vi "外观 1.vi"(0 "Data In":T6=enum."氨氮" caption="数据输入", 2 "Display State In":T3={"模块启用"={"环境动力"=FALSE, "氨氮"=FALSE, "总磷"=FALSE, "总氮"=FALSE, "高锰酸盐指数"=FALSE, "化学需氧量"=FALSE, "多参数"=FALSE, "加标回收"=FALSE, "GPS"=FALSE}, "模块名称"={"环境动力"="环境动力", "氨氮"="氨氮", "总磷"="总磷", "总氮"="总氮", "高锰酸盐指数"="高锰酸盐指数", "化学需氧量"="化学需氧量", "多参数"="多参数", "加标回收"="加标回收", "GPS"="GPS"}} caption="显示状态输入", 3 "Container State":T5 caption="容器状态") -> (6 "Data Out":T6=enum."氨氮" caption="数据输出", 7 "Display State Out":T3={"模块启用"={"环境动力"=FALSE, "氨氮"=FALSE, "总磷"=FALSE, "总氮"=FALSE, "高锰酸盐指数"=FALSE, "化学需氧量"=FALSE, "多参数"=FALSE, "加标回收"=FALSE, "GPS"=FALSE}, "模块名称"={"环境动力"="环境动力", "氨氮"="氨氮", "总磷"="总磷", "总氮"="总氮", "高锰酸盐指数"="高锰酸盐指数", "化学需氧量"="化学需氧量", "多参数"="多参数", "加标回收"="加标回收", "GPS"="GPS"}} caption="显示状态输出", 8 "Action":T2 caption="动作")   [LabVIEW 2016, in "运维调试菜单.xctl"]
uses:
  <vilib>/_xctls/Container State.ctl
  <vilib>/_xctls/Action.ctl
  <vilib>/Utility/miscctls.llb/LVPointTypeDef.ctl
  <vilib>/_xctls/XControlSupport.lvlib
panel:
  in  "单选按钮":T1
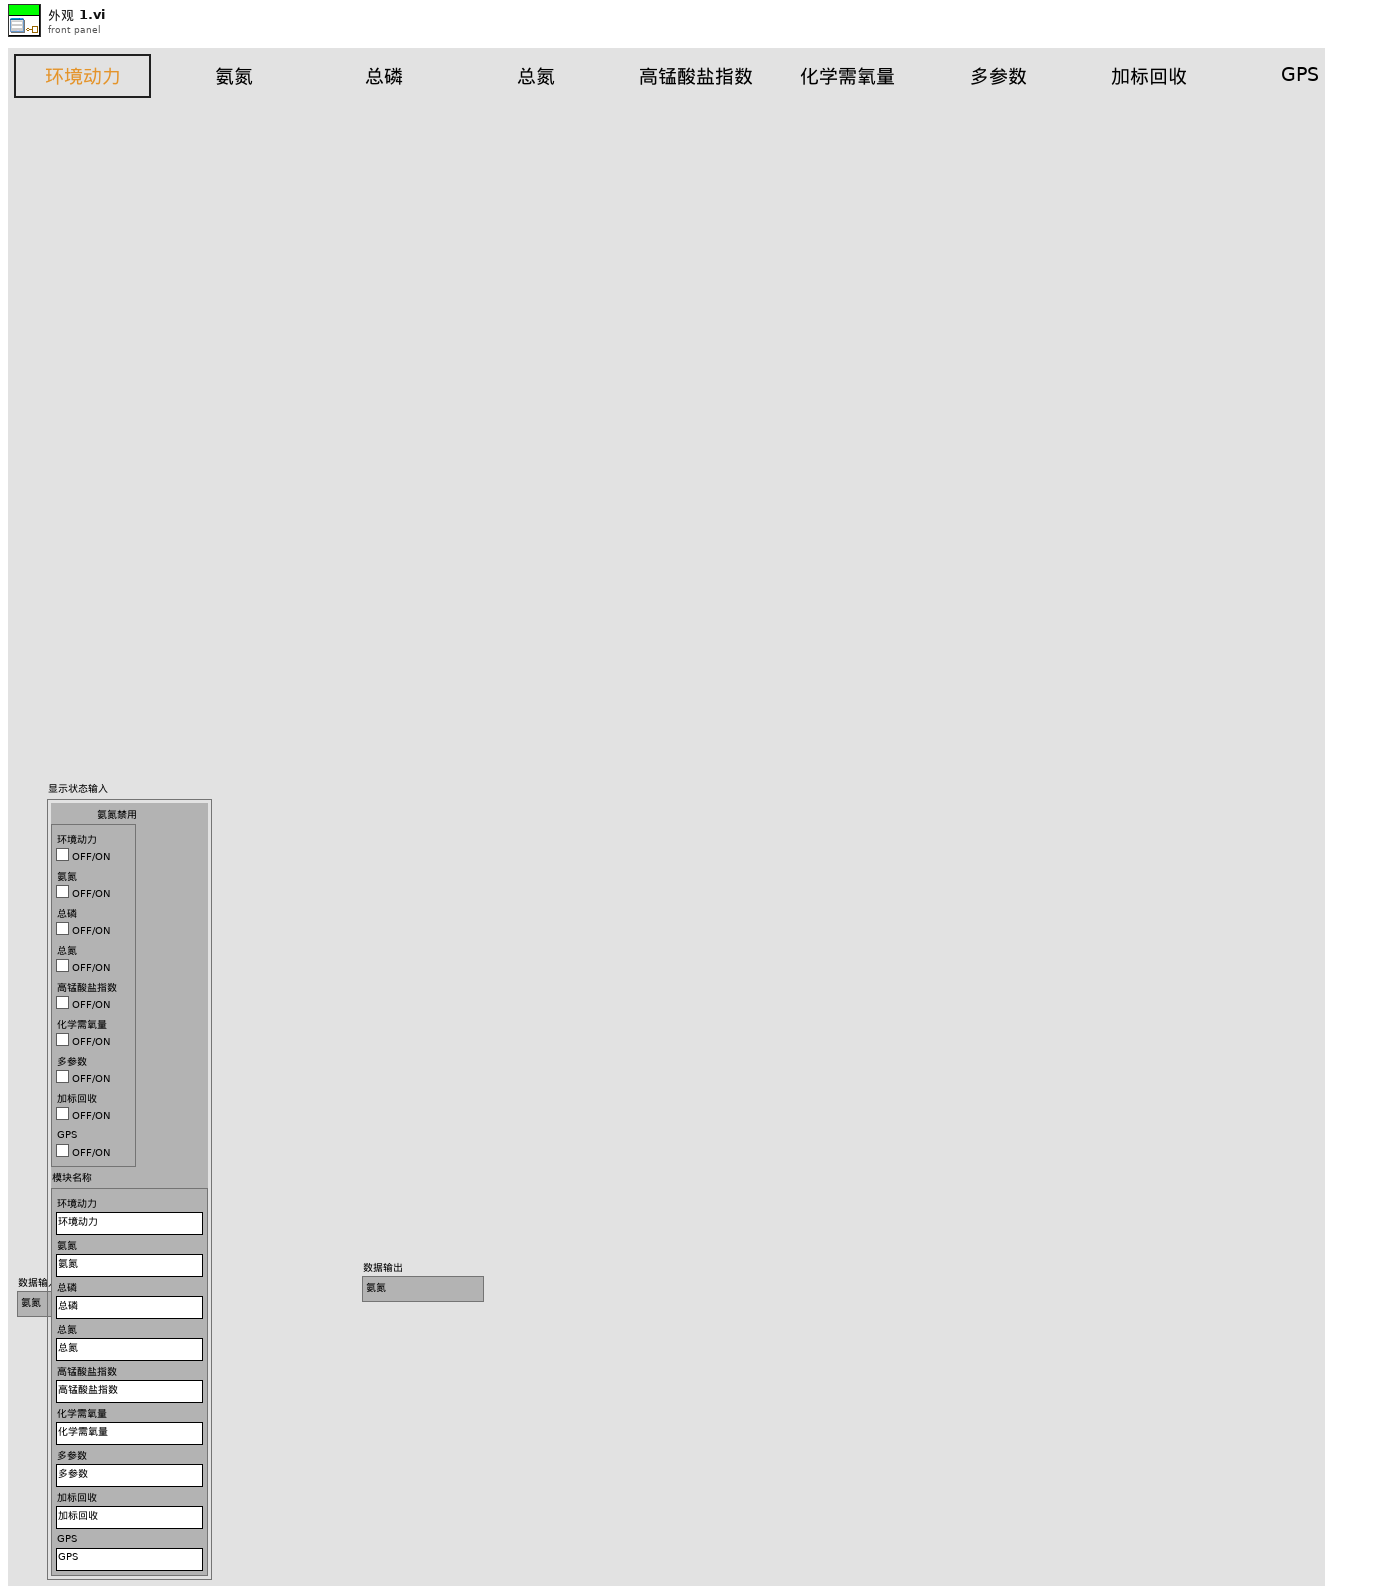
[diagram p1: front panel]
types:
  T1 = typedef "运维调试菜单.xctl/控件外观.ctl" = enum32{"环境动力", "氨氮", "总磷", "总氮", "高锰酸盐指数", "化学需氧量", "多参数", "加标回收", "GPS"}
  T2 = typedef "XControlSupport.lvlib/Action.ctl" = cluster{"Data Changed?":bool, "State Changed?":bool, "Action Name":string}
  T3 = typedef "运维调试菜单.xctl/状态 1.ctl" = cluster{"模块启用":T4, "模块名称":cluster{"环境动力":string, "氨氮":string, "总磷":string, "总氮":string, "高锰酸盐指数":string, "化学需氧量":string, "多参数":string, "加标回收":string, "GPS":string}}
  T4 = typedef "运维调试菜单.xctl/模块启用.ctl" = cluster{"环境动力":bool, "氨氮":bool, "总磷":bool, "总氮":bool, "高锰酸盐指数":bool, "化学需氧量":bool, "多参数":bool, "加标回收":bool, "GPS":bool}
  T5 = typedef "XControlSupport.lvlib/Container State.ctl" = cluster{"Indicator?":bool, "Run Mode?":bool, " Refnum":refnum<vi>}
  T6 = typedef "运维调试菜单.xctl/数据 1.ctl" = enum16{"环境动力", "氨氮", "总磷", "总氮", "高锰酸盐指数", "化学需氧量", "多参数", "加标回收", "GPS"}
  T7 = typedef "LVPointTypeDef.ctl" = cluster{"Horizontal":i16, "Vertical":i16}
  T8 = cluster{"环境动力":string, "氨氮":string, "总磷":string, "总氮":string, "高锰酸盐指数":string, "化学需氧量":string, "多参数":string, "加标回收":string, "GPS":string}
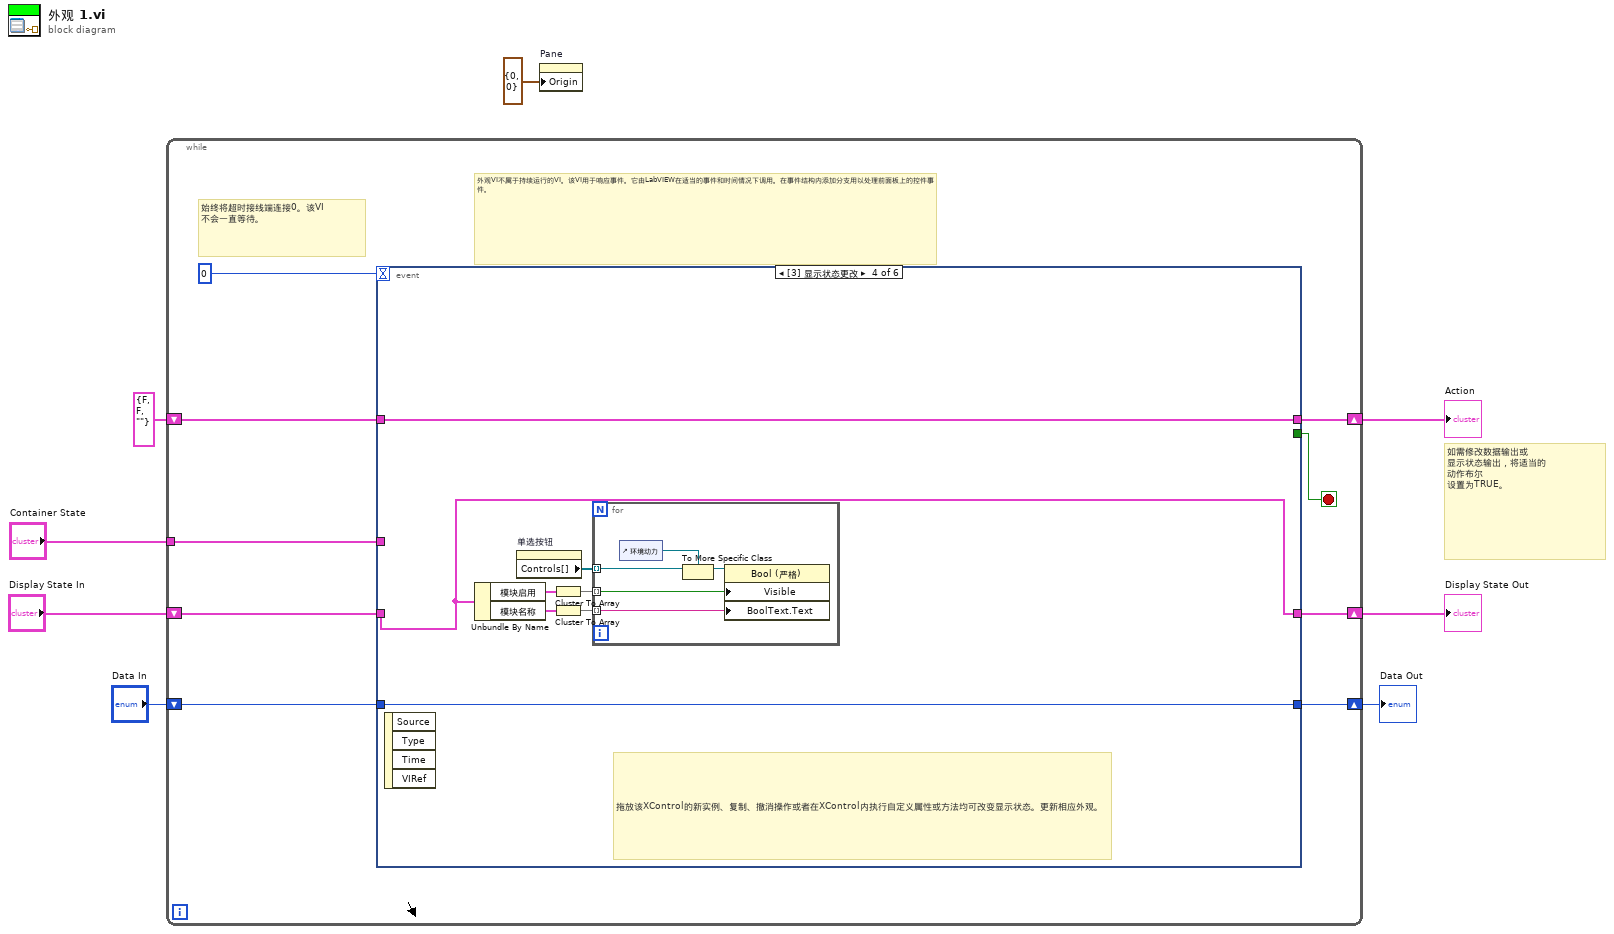
[diagram p0: block diagram]
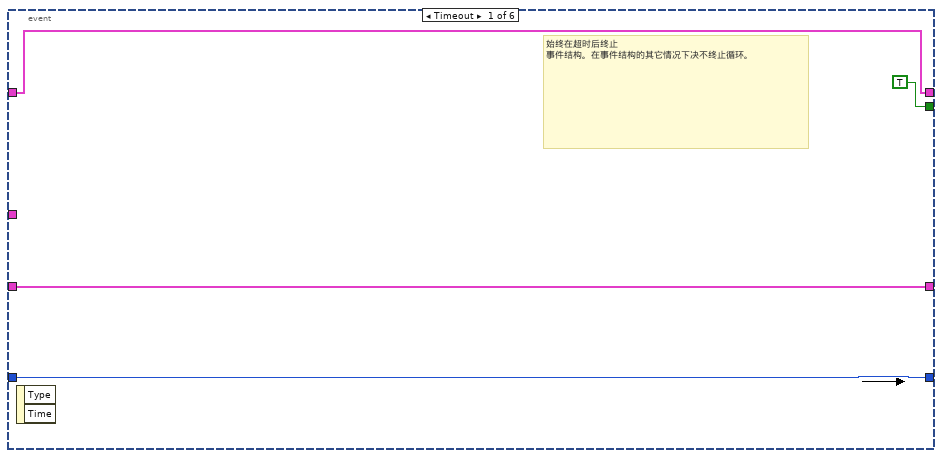
[diagram p2: hidden frame]
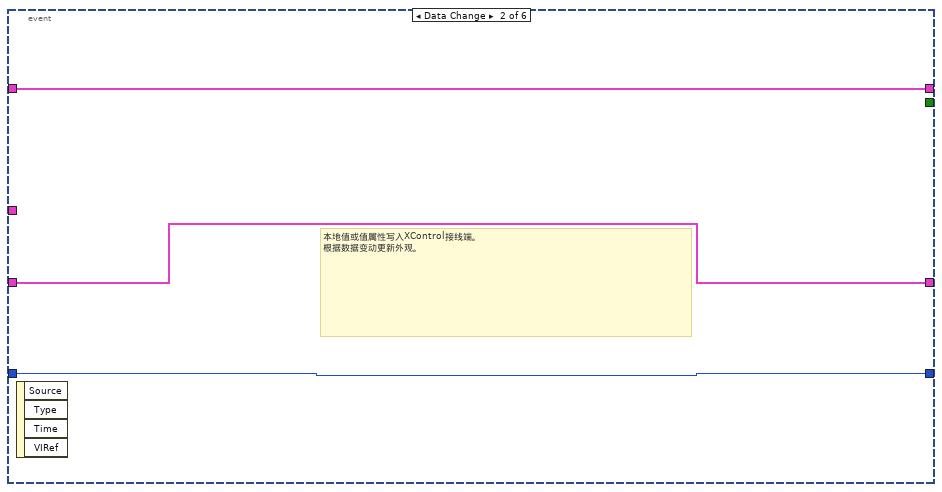
[diagram p3: hidden frame]
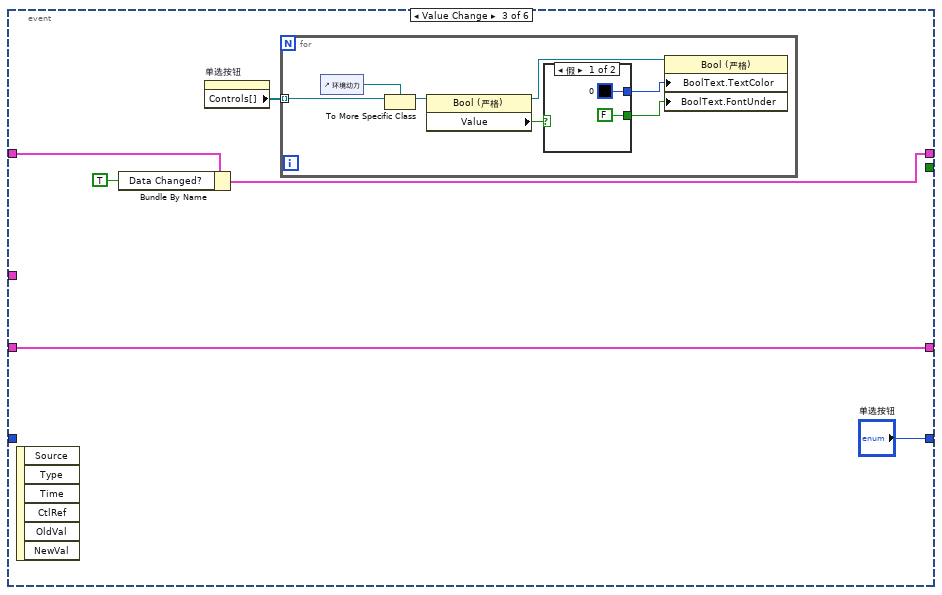
[diagram p4: hidden frame]
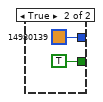
[diagram p5: hidden frame]
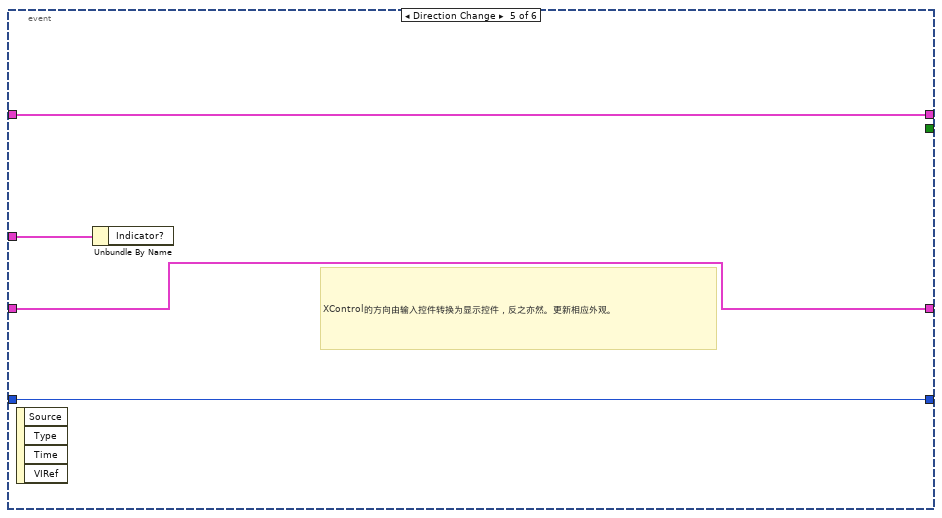
[diagram p6: hidden frame]
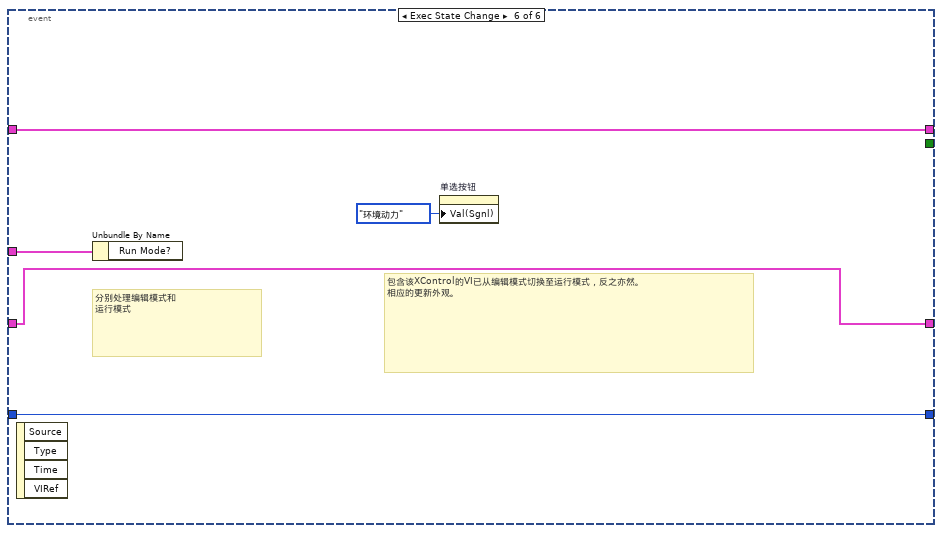
[diagram p7: hidden frame]
diagram:
  # "如需修改数据输出或\n显示状态输出，将适当的\n动作布尔\n设置为TRUE。"
  n1 = while {
    shift-right: [w16] -> w5
    shift-left: "Display State In" -> [w17]
    tunnel: "Container State" -> [w13]
    shift-right: [w11] -> w8
    shift-left: "Data In" -> [w12]
    shift-right: [w9] -> w3
    shift-left: T2 {"Data Changed?"=FALSE, "State Changed?"=FALSE, "Action Name"=""} ("Action") -> [w10]
    stop <- w15 stop-if-true
    # "外观VI不属于持续运行的VI。该VI用于响应事件。它由LabVIEW在适当的事件和时间情况下调用。在事件结构内添加分支用以处理前面板上的控件事件。"
    # "始终将超时接线端连接0。该VI\n不会一直等待。"
    n2 = event shown="[3] 显示状态更改" {
      selector: _ -> [_ _ _ _ _ _]
      dyn-events: _ -> [_ _ _ _ _ _]
      timeout: 0 -> [_ _ _ _ _ _]
      tunnel: w17 -> [w19 w23 w30 w47 w57 w62]
      tunnel: [w19 w23 w30 w47 w57 w62] -> w16
      tunnel: [TRUE _ _ _ _ _] -> w15
      tunnel: w13 -> [_ _ _ _ w58 w63]
      tunnel: w12 -> [w18 w24 _ w49 w56 w61]
      tunnel: [w18 w24 "单选按钮" w49 w56 w61] -> w11
      tunnel: [w20 w22 w28 w48 w55 w60] -> w9
      tunnel: w10 -> [w20 w22 w29 w48 w55 w60]
      event Timeout {
        # "始终在超时后终止\n事件结构。在事件结构的其它情况下决不终止循环。"
        n3 = event-data() -> ()  [unwired: 1 in, 2 out]
      }
      event Data Change {
        # "本地值或值属性写入XControl接线端。\n根据数据变动更新外观。"
        n4 = event-data() -> ()  [unwired: 1 in, 4 out]
      }
      event Value Change {
        n5 = event-data() -> ()  [unwired: 1 in, 6 out]
        n6 = Bundle By Name(cluster=w29, "Data Changed?"=TRUE) -> (w28:T2)
        n7 = property on="单选按钮" class="RadioBtnsControl (严格)"() -> ("Controls[]"=w26:refnum<vi>[])  [unwired: 2 in, 2 out]
        n8 = for {
          tunnel: w26 -> [w37] mode=indexing
          n9 = control-ref of="环境动力"() -> (w31:refnum<vi>)
          n10 = To More Specific Class(target class=w31, reference=w37) -> (specific class reference=w36:refnum<vi>)  [unwired: 1 in, 1 out]
          n11 = property class="Bool (严格)"(reference=w36) -> (reference out=w35:refnum<vi>, "Value"=w34:bool)  [unwired: 1 in, 1 out]
          n12 = case shown="假" w34 {
            tunnel: [u32 0 u32 14980139] -> w33
            tunnel: [FALSE ("布尔文本.字体:下划线") TRUE ("布尔文本.字体:下划线")] -> w32
            frame False {
            }
            frame True {
            }
          }
          n13 = property class="Bool (严格)"(reference=w35, "BoolText.TextColor"=w33, "BoolText.FontUnder"=w32) -> ()  [unwired: 1 in, 2 out]
        }
      }
      event Display State Change {
        # "拖放该XControl的新实例、复制、撤消操作或者在XControl内执行自定义属性或方法均可改变显示状态。更新相应外观。"
        n14 = event-data() -> ()  [unwired: 1 in, 4 out]
        n15 = Unbundle By Name(w47) -> ("模块启用"=w45:T4, "模块名称"=w43:T8)
        n16 = property on="单选按钮" class="RadioBtnsControl (严格)"() -> ("Controls[]"=w46:refnum<vi>[])  [unwired: 2 in, 2 out]
        n17 = Cluster To Array(cluster=w45) -> (array=w44:bool[])
        n18 = Cluster To Array(cluster=w43) -> (array=w42:string[])
        n19 = for {
          tunnel: w46 -> [w54] mode=indexing
          tunnel: w44 -> [w51] mode=indexing
          tunnel: w42 -> [w50] mode=indexing
          n20 = control-ref of="环境动力"() -> (w52:refnum<vi>)
          n21 = To More Specific Class(target class=w52, reference=w54) -> (specific class reference=w53:refnum<vi>)  [unwired: 1 in, 1 out]
          n22 = property class="Bool (严格)"(reference=w53, "Visible"=w51, "BoolText.Text"=w50) -> ()  [unwired: 1 in, 2 out]
        }
      }
      event Direction Change {
        # "XControl的方向由输入控件转换为显示控件，反之亦然。更新相应外观。"
        n23 = event-data() -> ()  [unwired: 1 in, 4 out]
        n24 = Unbundle By Name(w58) -> ()  [unwired: 1 out]
      }
      event Exec State Change {
        # "包含该XControl的VI已从编辑模式切换至运行模式，反之亦然。\n相应的更新外观。"
        # "分别处理编辑模式和\n运行模式"
        n25 = event-data() -> ()  [unwired: 1 in, 4 out]
        n26 = Unbundle By Name(w63) -> ()  [unwired: 1 out]
        n27 = property on="单选按钮" class="RadioBtnsControl (严格)"("Val(Sgnl)"=控件外观."环境动力" ("值(信号)")) -> ()  [unwired: 2 in, 2 out]
      }
    }
  }
  "Display State Out" <- w5
  "Data Out" <- w8
  "Action" <- w3
  n28 = property on="Pane" class="Pane"("Origin"=T7 {"Horizontal"=0, "Vertical"=0} ("原点")) -> ()  [unwired: 2 in, 2 out]
